vi "Move Sequence.vi"(8 "Distance Up":dbl=28.0, 11 "Distance Down":dbl=28.0) -> ()   [LabVIEW 2014]
uses:
  Begin/Global Variables.vi
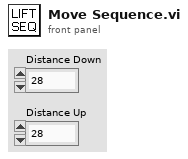
[diagram p1: front panel]
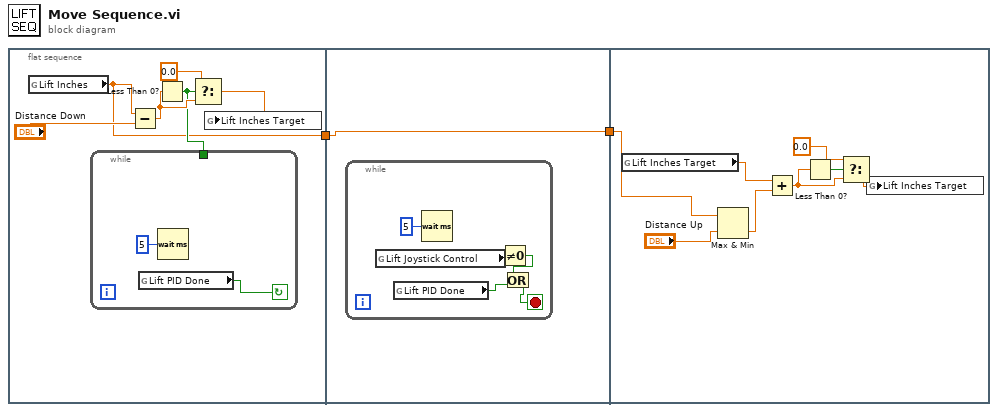
[diagram p0: block diagram]
diagram:
  n1 = flat-sequence {
    tunnel: [w3] -> w1
    tunnel: [w11] -> w2
    tunnel: w1 -> [w11]
    tunnel: w2 -> [w17]
    frame #0 {
      n2 = global read "Global Variables.vi" "Lift Inches"() -> (w3:dbl)
      n3 = Subtract(x=w3, y="Distance Down") -> (x-y=w7:dbl)
      n4 = Less Than 0?(x=w7) -> (x < 0?=w4:bool)
      n5 = while {
        tunnel: w4 -> [_]
        stop <- w9 continue-if-true
        n6 = global read "Global Variables.vi" "Lift PID Done"() -> (w9:bool)
        n7 = Wait (ms)(milliseconds to wait=u32 5) -> ()  [unwired: 1 out]
      }
      n8 = Select(t=0.0, s=w4, f=w7) -> (s? t:f=w6:dbl)
      n9 = global write "Global Variables.vi" "Lift Inches Target"(w6) -> ()
    }
    frame #1 {
      n10 = while {
        stop <- w12 stop-if-true
        n11 = global read "Global Variables.vi" "Lift Joystick Control"() -> (w14:dbl)
        n12 = global read "Global Variables.vi" "Lift PID Done"() -> (w15:bool)
        n13 = Wait (ms)(milliseconds to wait=u32 5) -> ()  [unwired: 1 out]
        n14 = Not Equal To 0?(x=w14) -> (x != 0?=w13:bool)
        n15 = Or(x=w13, y=w15) -> (x .or. y?=w12:bool)
      }
    }
    frame #2 {
      n16 = global read "Global Variables.vi" "Lift Inches Target"() -> (w22:dbl)
      n17 = Max & Min(x=w17, y="Distance Up") -> (min(x,y)=w18:dbl)  [unwired: 1 out]
      n18 = Add(x=w22, y=w18) -> (x+y=w23:dbl)
      n19 = Less Than 0?(x=w23) -> (x < 0?=w24:bool)
      n20 = Select(t=0.0, s=w24, f=w23) -> (s? t:f=w21:dbl)
      n21 = global write "Global Variables.vi" "Lift Inches Target"(w21) -> ()
    }
  }
